vi "GRADING - Copy (2).vi"() -> ()   [LabVIEW 2025]
panel:
  out "FAIL":bool
  out "GRADE C":bool
  out "GRADE B":bool
  out "GRADE A":bool
  in  "MARKS":dbl
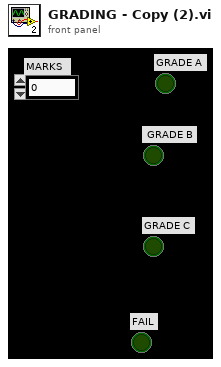
[diagram p1: front panel]
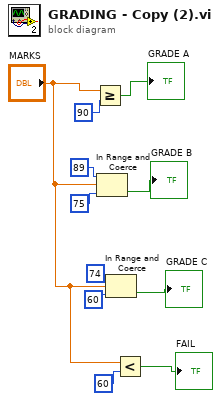
[diagram p0: block diagram]
diagram:
  n1 = Greater Or Equal?(x="MARKS", y=90) -> (x >= y?=→"GRADE A":bool)
  n2 = In Range and Coerce(upper limit=89, x="MARKS", lower limit=75) -> (In Range?=→"GRADE B":bool)  [unwired: 1 out]
  n3 = In Range and Coerce(upper limit=74, x="MARKS", lower limit=60) -> (In Range?=→"GRADE C":bool)  [unwired: 1 out]
  n4 = Less?(x="MARKS", y=60) -> (x < y?=→"FAIL":bool)
